vi "Get flattened data.vi"(8 "error in (no error)":errorcluster, 11 "U32 D Element in":refnum<class "U32 D Element.lvclass">) -> (0 "error out":errorcluster, 2 "Flattened data":u8[](array[numeric]), 3 "U32 D Element out":refnum<class "U32 D Element.lvclass">)   [LabVIEW 2018, in "D Datagrid Library.lvlib" / "U32 D Element.lvclass"]
uses:
  U32 D Element.lvclass
  U32 D Element.lvclass/U32 D Element.ctl
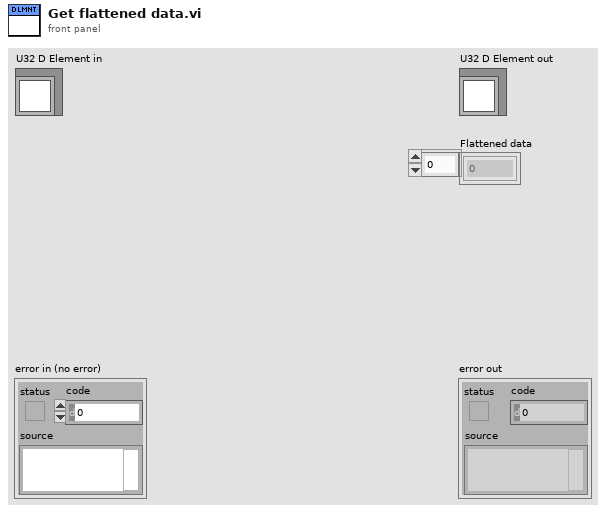
[diagram p1: front panel]
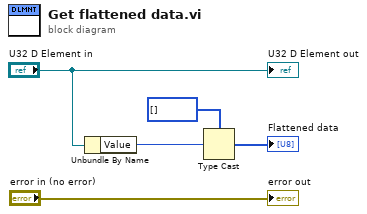
[diagram p0: block diagram]
diagram:
  n1 = Unbundle By Name("U32 D Element in") -> ("Value"=w1:u32)
  n2 = Type Cast(type=u8[] [] ("Flattened data"), x=w1) -> (*(type *) &x=→"Flattened data":u8[])
  "error out" <- "error in (no error)"
  "U32 D Element out" <- "U32 D Element in"
